vi "Shutdown Shield.vi"(8 "error in (no error)":errorcluster, 11 "Wi-Fi Shield in":refnum<class "Wi-Fi Shield.lvclass">) -> (0 "error out":errorcluster, 3 "Wi-Fi Shield out":refnum<class "Wi-Fi Shield.lvclass">)   [LabVIEW 2020, in "Wi-Fi Shield.lvclass"]
uses:
  Wi-Fi Shield.lvclass
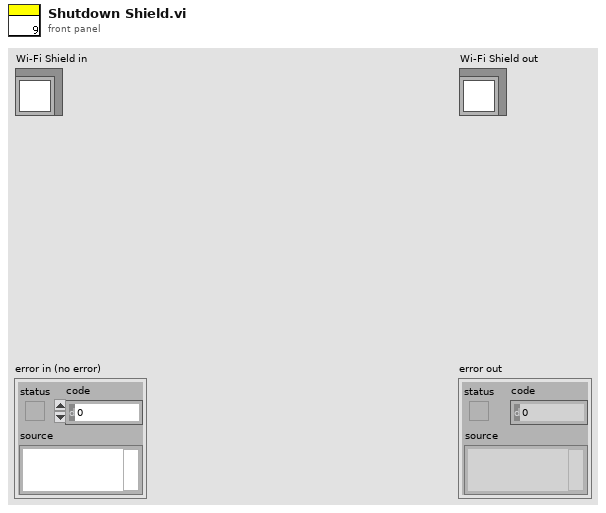
[diagram p1: front panel]
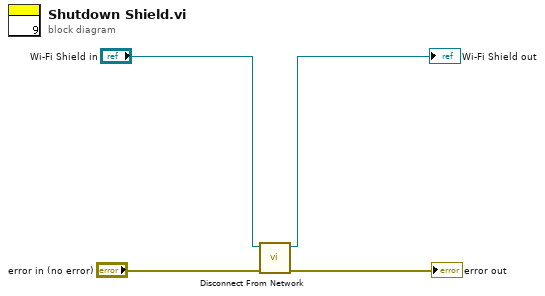
[diagram p0: block diagram]
diagram:
  n1 = call-dynamic "Disconnect From Network.vi"("error in (no error)"="error in (no error)", "Wi-Fi Shield in"="Wi-Fi Shield in") -> ("error out"=→"error out":errorcluster, "Wi-Fi Shield out"=→"Wi-Fi Shield out":refnum<class "Wi-Fi Shield.lvclass">)  [unwired: 8 in]
